vi "Demote Element (EXT).vi"(9 "Index to Demote":i32, 11 "Array In":ext[](array[numeric])) -> (3 "Array Out":ext[](array[numeric]))   [LabVIEW 2015, in "ArrayExtensions.lvlib"]
uses:
  ArrayExtensions.lvlib
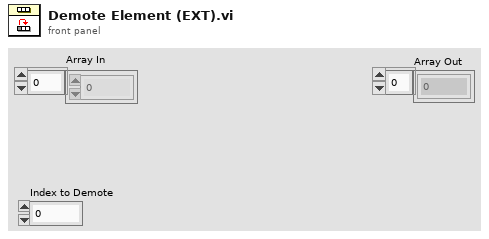
[diagram p1: front panel]
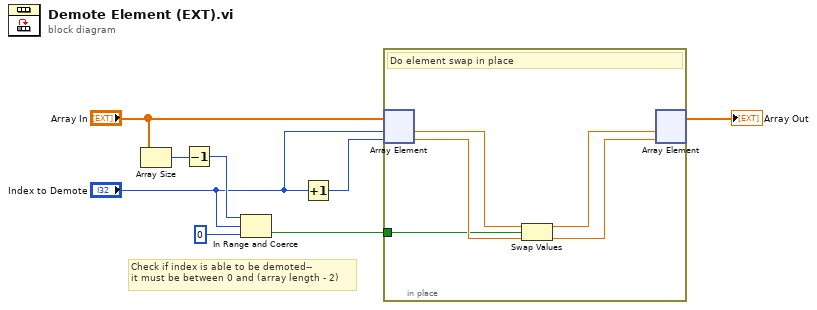
[diagram p0: block diagram]
diagram:
  # "Check if index is able to be demoted--\nit must be between 0 and (array length - 2)"
  n1 = Array Size(array="Array In") -> (size(s)=w5:i32)
  n2 = Decrement(x=w5) -> (x-1=w3:i32)
  n3 = In Range and Coerce(upper limit=w3, x="Index to Demote", lower limit=0) -> (In Range?=w4:bool)  [unwired: 1 out]
  n4 = Increment(x="Index to Demote") -> (x+1=w1:i32)
  n5 = in-place {
    in-place-border: w4 -> [w9]
    # "Do element swap in place"
    n6 = in-place-array #1("Array In", "Index to Demote", w1) -> (w13:ext, w12:ext)
    n7 = Swap Values(12:w13, 13:w9, 14:w12) -> (1:w11:ext, 3:w10:ext)
    n8 = in-place-array #1(w11, w10) -> (→"Array Out":ext[])  [unwired: 2 out]
  }
